vi "MainFPGA.vi"() -> ()   [LabVIEW 2016]
uses:
  <vilib>/rvi/Emulation/niFpgaGetClockAttributes.vi
  <vilib>/rvi/Emulation/niFpgaSctlEmulationGetInTimedLoop.vi
  <vilib>/rvi/Emulation/niFpgaEmulationReportErrorSimple.vi
  <vilib>/rvi/interface/RandomDataEmulation/nirviRandomDataMultiElementFPGAFIFO.vi
  <instcachedir>/0/nirviRandomDataMultiElementFPGAFIFO_6740B454F3C245F78F76ED91F73FD8DB.lvgen/nirviRandomDataMultiElementFPGAFIFO_6740B454F3C245F78F76ED91F73FD8DB_001.vi
  <vilib>/rvi/interface/RandomDataEmulation/niFpgaRandomDataHandleErrors.vi
  <vilib>/rvi/eio/common/nirviEmuTemplateMethod_errors.vi
  <vilib>/rvi/Emulation/niFpgaCriticalErrorInLSC.vi
  <vilib>/rvi/DataTransferAndStorage/Container/XNode/niFpgaContainer.xnode
  <vilib>/rvi/interface/RandomDataEmulation/nirviRandomDataFpgaMultiElementTemplate.vi
  <vilib>/eio/EIONode/EIONode.xnode
panel:
  out "Ch1":fxp<+/-,20,5>
  out "Ch0":fxp<+/-,20,5>
  out "Ch1 < 0?":bool
  out "Ch1 > 10?":bool
  out "Ch0 < 0?":bool
  out "Ch0 >10?":bool
  in  "stop":bool
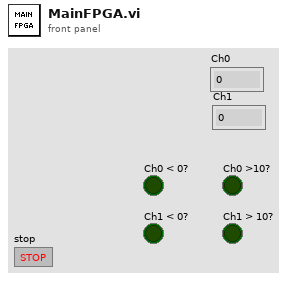
[diagram p1: front panel]
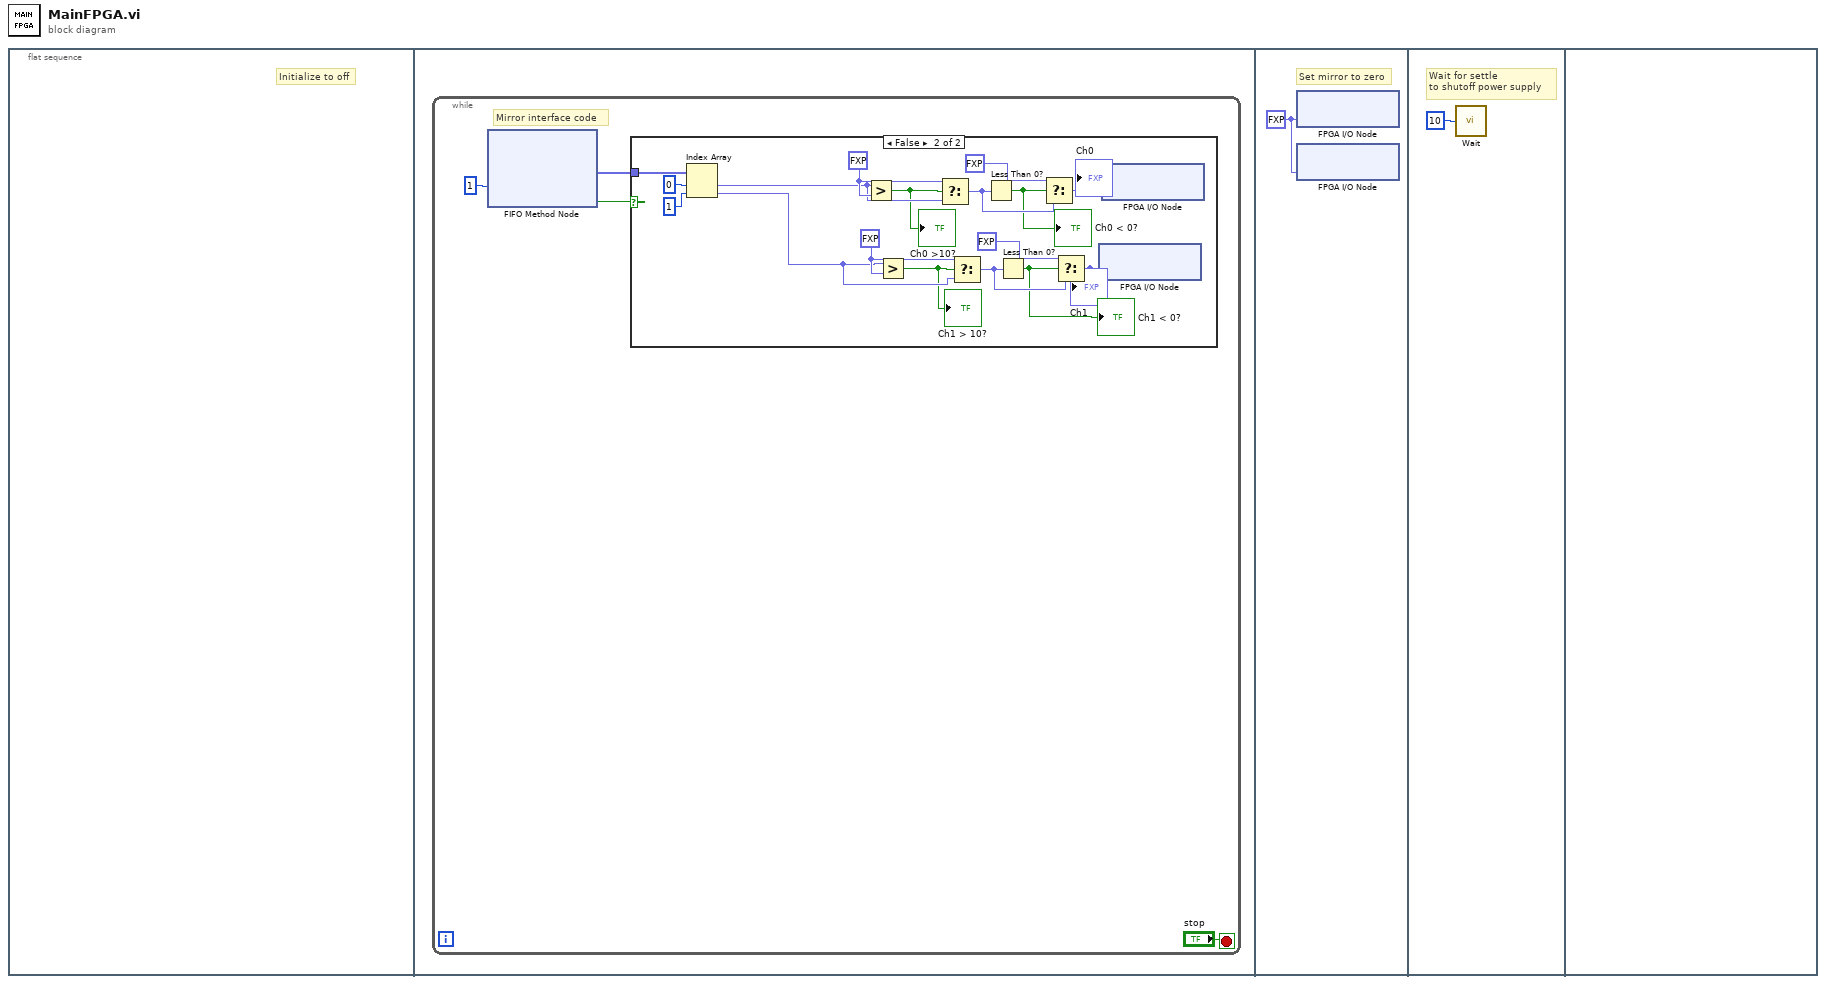
[diagram p0: block diagram]
diagram:
  n1 = flat-sequence {
    frame #0 {
      # "Initialize to off"
    }
    frame #1 {
      n2 = while {
        stop <- "stop" stop-if-true
        # "Mirror interface code"
        n3 = xnode ("FIFO Method Node")("Timeout"=1) -> ("Element"=w1:fxp<+/-,20,5>[], "Timed Out?"=w2:bool)  [unwired: 1 in, 1 out]
        n4 = case shown="False" w2 {
          tunnel: w1 -> [_ w21]
          frame True {
          }
          frame False {
            w13 = fxp<+/-,20,5> 10.0 ("y")
            w18 = fxp<+/-,20,5> 10.0 ("y")
            n5 = Index Array(array=w21, index #1=0 ("index"), index #2=1 ("length")) -> (element #1=w17:fxp<+/-,20,5>, element #2=w9:fxp<+/-,20,5>)
            n6 = Greater?(x=w17, y=w18) -> (0:w6:bool)
            "Ch0 >10?" <- w6
            n7 = Greater?(x=w9, y=w13) -> (0:w7:bool)
            "Ch1 > 10?" <- w7
            n8 = Select(t=w18, s=w6, f=w17) -> (s? t:f=w16:fxp<+/-,20,5>)
            n9 = Select(t=w13, s=w7, f=w9) -> (s? t:f=w12:fxp<+/-,20,5>)
            n10 = Less Than 0?(x=w16) -> (x < 0?=w5:bool)
            "Ch0 < 0?" <- w5
            n11 = Less Than 0?(x=w12) -> (x < 0?=w8:bool)
            "Ch1 < 0?" <- w8
            n12 = Select(t=fxp<+/-,20,5> 0.0, s=w5, f=w16) -> (s? t:f=w14:fxp<+/-,20,5>)
            "Ch0" <- w14
            n13 = Select(t=fxp<+/-,20,5> 0.0, s=w8, f=w12) -> (s? t:f=w10:fxp<+/-,20,5>)
            "Ch1" <- w10
            n14 = xnode "FPGA I/O Node"("Mod5/AO1"=w10) -> ()  [unwired: 1 in, 1 out]
            n15 = xnode "FPGA I/O Node"("Mod5/AO0"=w14) -> ()  [unwired: 1 in, 1 out]
          }
        }
      }
    }
    frame #2 {
      w22 = fxp<+/-,20,5> 0.0 ("Mod5/AO2")
      # "Set mirror to zero"
      n16 = xnode "FPGA I/O Node"("Mod5/AO0"=w22) -> ()  [unwired: 1 in, 1 out]
      n17 = xnode "FPGA I/O Node"("Mod5/AO1"=w22) -> ()  [unwired: 1 in, 1 out]
    }
    frame #3 {
      # "Wait for settle \nto shutoff power supply"
      n18 = call "Wait"("Count(mSec)"=u32 10) -> ()  [unwired: 1 out]
    }
    frame #4 {
    }
  }
